vi "CreateFileIVPath.vi"(8 "error in 2":errorcluster, 11 "DAQ File Name":string) -> (0 "error out 2":errorcluster, 3 "appended path 2":path)   [LabVIEW 2019, in "SMU.lvclass"]
uses:
  SMU.lvclass
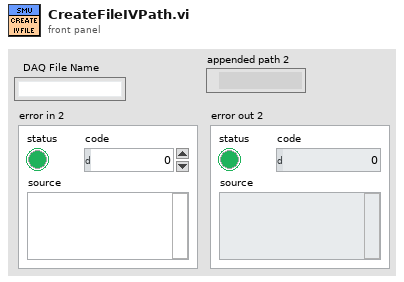
[diagram p1: front panel]
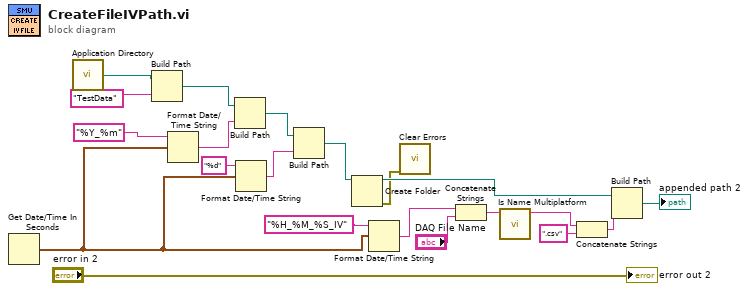
[diagram p0: block diagram]
diagram:
  n1 = Get Date/Time In Seconds() -> (seconds since 1Jan1904=w7:timestamp)
  n2 = call <vilib>:"Application Directory.vi"() -> ("Application Directory"=w18:path)
  n3 = Build Path(base path=w18, name or relative path="TestData") -> (appended path=w9:path)
  n4 = Format Date/Time String(time format string (%c)="%Y_%m", seconds (now)=w7) -> (date/time string=w10:string)  [unwired: 1 in]
  n5 = Build Path(base path=w9, name or relative path=w10) -> (appended path=w8:path)
  n6 = Format Date/Time String(time format string (%c)="%d", seconds (now)=w7) -> (date/time string=w5:string)  [unwired: 1 in]
  n7 = Build Path(base path=w8, name or relative path=w5) -> (appended path=w4:path)
  n8 = Create Folder(path (use dialog)=w4) -> (created path=w15:path, error out=w14:errorcluster)  [unwired: 2 in, 1 out]
  n9 = Format Date/Time String(time format string (%c)="%H_%M_%S_IV", seconds (now)=w7) -> (date/time string=w20:string)  [unwired: 1 in]
  n10 = call <vilib>:"Clear Errors.vi"("error in (no error)"=w14) -> ()  [unwired: 5 in, 2 out]
  n11 = Concatenate Strings(w20, "DAQ File Name") -> (w16:string)
  n12 = call <vilib>:"Is Name Multiplatform.vi"("filename"=w16) -> ("suggested filename"=w2:string)  [unwired: 6 in, 4 out]
  n13 = Concatenate Strings(w2, ".csv" ("string")) -> (w1:string)
  n14 = Build Path(base path=w15, name or relative path=w1) -> (appended path=→"appended path 2":path)
  "error out 2" <- "error in 2"
